vi "CSTK_MCListbox_Designer_DeleteColHdr.vi"(7 "表头属性列表输入":refnum<vi>, 8 "错误输入（无错误）":errorcluster, 9 "Selected Index":i32, 10 "MCListbox引用句柄":refnum<vi>, 11 "VI输入":refnum<vi>) -> (0 "错误输出":errorcluster, 3 "VI输出":refnum<vi>)   [LabVIEW 2015, in "CSTK_MCListbox Designer.lvlib"]
uses:
  CSTK_MCListbox Designer.lvlib
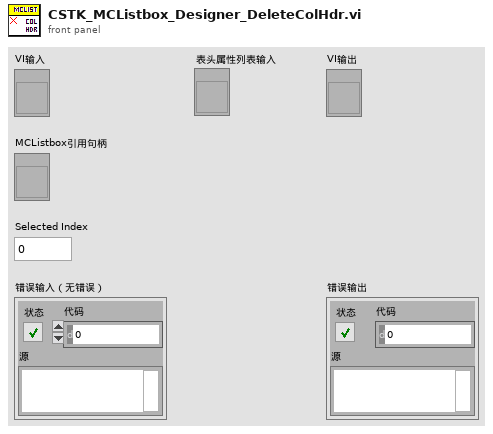
[diagram p1: front panel]
types:
  T1 = typedef "CSTK_MCListbox Designer.lvlib/_CSTK_MCListbox_Designer_ColHdr_Selected.ctl" = cluster{"选择":bool, "表头属性":T2}
  T2 = typedef "CSTK_MCListbox Designer.lvlib/_CSTK_MCListbox_Designer_ColHdr.ctl" = cluster{"列名称":string, "单元格宽度":u32, "粗体":bool, "斜体":bool, "对齐":enum16{"Left", "Center", "Right"}}
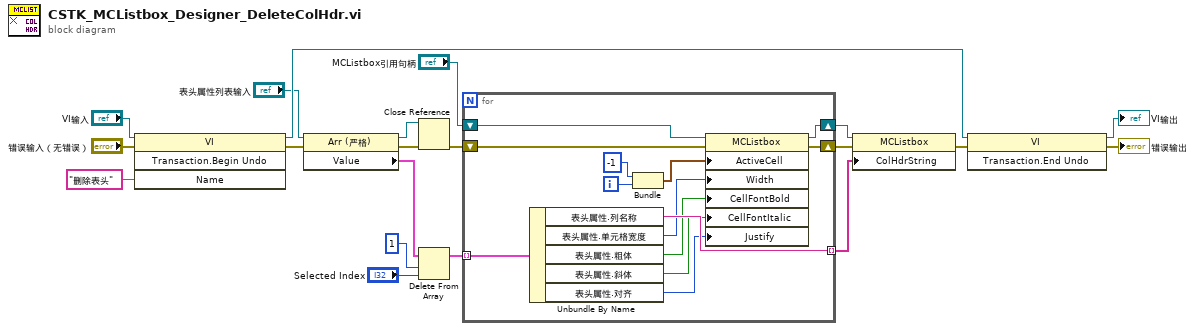
[diagram p0: block diagram]
diagram:
  n1 = invoke class="VI" method="Transaction.Begin Undo"(reference="VI输入", error in="错误输入（无错误）", "Name"="删除表头" ("名称")) -> (reference out=w5:refnum<vi>, error out=w14:errorcluster)  [unwired: 1 in, 2 out]
  n2 = property on="属性节点" class="Arr (严格)"(reference="表头属性列表输入", error in=w14) -> (reference out=w3:refnum<vi>, error out=w4:errorcluster, "Value"=w15:T1[])
  n3 = Close Reference(reference=w3, error in (no error)=w4) -> (error out=w2:errorcluster)
  n4 = Delete From Array(array=w15, length=1 ("长度"), index="Selected Index") -> (array with subset deleted=w16:T1[])  [unwired: 1 out]
  n5 = for {
    tunnel: w16 -> [w31] mode=indexing
    tunnel: [w30] -> w19 mode=indexing
    shift-right: [w27] -> w17
    shift-left: "MCListbox引用句柄" -> [w28]
    shift-right: [w22] -> w18
    shift-left: w2 -> [w23]
    i -> [w32]
    n6 = Unbundle By Name(w31) -> ("表头属性.列名称"=w30:string, "表头属性.单元格宽度"=w26:u32, "表头属性.粗体"=w25:bool, "表头属性.斜体"=w21:bool, "表头属性.对齐"=w24:enum16{"Left", "Center", "Right"})
    n7 = Bundle(-1, w32) -> (w29:cluster{i32, i32})  [unwired: 1 in]
    n8 = property class="MCListbox"(reference=w28, error in=w23, "ActiveCell"=w29, "Width"=w26, "CellFontBold"=w25, "CellFontItalic"=w21, "Justify"=w24) -> (reference out=w27:refnum<vi>, error out=w22:errorcluster)
  }
  n9 = property class="MCListbox"(reference=w17, error in=w18, "ColHdrString"=w19) -> (error out=w20:errorcluster)  [unwired: 1 out]
  n10 = invoke class="VI" method="Transaction.End Undo"(reference=w5, error in=w20) -> (reference out=→"VI输出":refnum<vi>, error out=→"错误输出":errorcluster)  [unwired: 1 in, 1 out]
